vi "DAQ.vi"(0 "sample length":i32=100, 5 "task/channels in":refnum<k21>, 7 "SetVoltage":dbl=3.3 format="%#_13g", 9 "error in":errorcluster, 11 "VISA resource name out":refnum<visa-resource-name>, 12 "error out":errorcluster) -> (4 "task out":refnum<k21>, 6 "error out 2":errorcluster, 10 "VISA resource name out 2":refnum<visa-resource-name>, 15 "error out 3":errorcluster)   [LabVIEW 2018]
uses:
  <vilib>/DAQmx/read.llb/DAQmx Read (Analog DBL 1Chan 1Samp).vi
  GlobalVariables/GlobalStop.vi
  GlobalVariables/SetVoltagGlobal.vi
  GlobalVariables/Voltage Level Global.vi
  GlobalVariables/CurrentLevelGlobal.vi
  <vilib>/DAQmx/miscellaneous.llb/DAQmx Fill In Error Info.vi
  GlobalVariables/WaveformCharGlobal.vi
  <vilib>/ptbypt/NI_PtbyPt.lvlib
  OriginalCodeFolder/C/Program Files (x86)/National Instruments/LabVIEW 2018/instr.lib/XP Power PLS600/XP Power PLS600.lvlib
panel:
  in  "Over Voltage\nProtection":dbl=300.0 format="%#_13g"
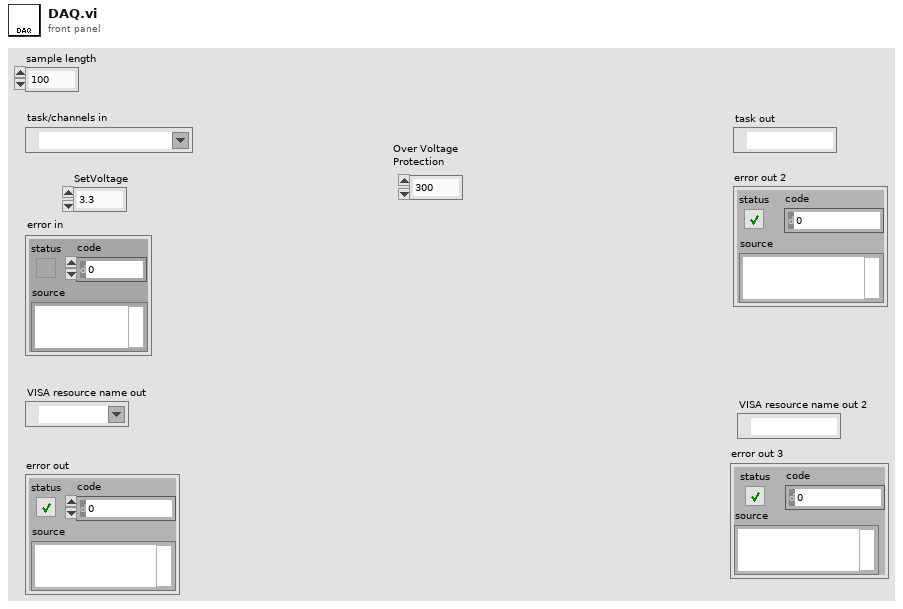
[diagram p1: front panel]
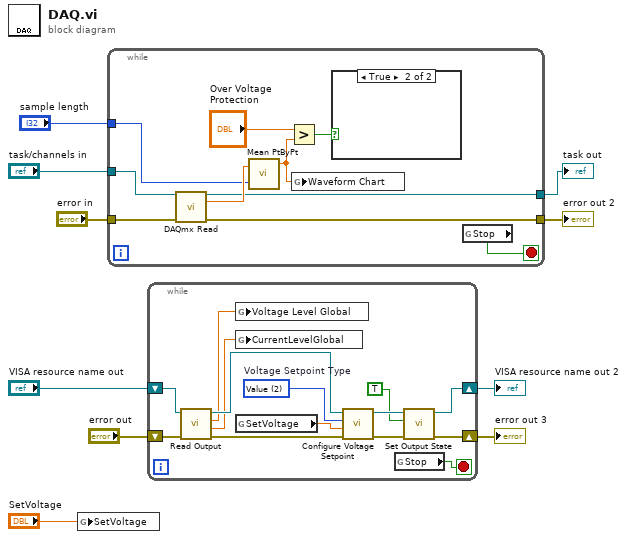
[diagram p0: block diagram]
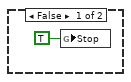
[diagram p2: hidden frame]
diagram:
  n1 = global write "SetVoltagGlobal.vi" "SetVoltage"("SetVoltage") -> ()
  n2 = while {
    tunnel: "sample length" -> [w14]
    tunnel: "task/channels in" -> [w13]
    tunnel: [w19] -> w3
    tunnel: "error in" -> [w12]
    tunnel: [w18] -> w4
    stop <- w15 stop-if-true
    n3 = call-poly <vilib>:"DAQmx Read.vi"("task/channels in"=w13, "error in"=w12) -> ("task out"=w19:refnum<k21>, "data"=w20:dbl, "error out"=w18:errorcluster)  [unwired: 11 in]
    n4 = call <vilib>:"Mean PtByPt.vi"("x"=w20, "sample length"=w14) -> ("mean"=w11:dbl)  [unwired: 2 in, 1 out]
    n5 = Greater?(x="Over Voltage\nProtection", y=w11) -> (0:w17:bool)
    n6 = global write "WaveformCharGlobal.vi" "Waveform Chart"(w11) -> ()
    n7 = case shown="True" w17 {
      frame False {
        n8 = global write "GlobalStop.vi" "Stop"(TRUE ("Over Allowable\nVoltage")) -> ()
      }
      frame True {
      }
    }
    n9 = global read "GlobalStop.vi" "Stop"() -> (w15:bool)
  }
  "error out 2" <- w4
  "task out" <- w3
  n10 = while {
    shift-right: [w31] -> w1
    shift-left: "error out" -> [w29]
    shift-right: [w30] -> w2
    shift-left: "VISA resource name out" -> [w27]
    stop <- w25 stop-if-true
    w33 = 2 items=["Minimum", "Maximum", "Value"]  # Voltage Setpoint Type
    n11 = call "Read Output.vi"("error in (no error)"=w29, "VISA resource name"=w27) -> ("error out"=w28:errorcluster, "Actual Current Level (amperes)"=w22:dbl, "Actual Voltage Level (volts)"=w23:dbl, "VISA resource name out"=w26:refnum<visa-resource-name>)  [unwired: 6 in]
    n12 = global write "Voltage Level Global.vi" "Voltage Level Global"(w23) -> ()
    n13 = global write "CurrentLevelGlobal.vi" "CurrentLevelGlobal"(w22) -> ()
    n14 = global read "SetVoltagGlobal.vi" "SetVoltage"() -> (w24:dbl)
    n15 = call "Configure Voltage Setpoint.vi"("error in (no error)"=w28, "Voltage Setpoint (0 volts)"=w24, "Voltage Setpoint Type (0: Minimum)"=w33, "VISA resource name"=w26) -> ("error out"=w34:errorcluster, "VISA resource name out"=w35:refnum<visa-resource-name>)  [unwired: 6 in]
    n16 = global read "GlobalStop.vi" "Stop"() -> (w25:bool)
    n17 = call "Set Output State.vi"("error in (no error)"=w34, "Output State (F: Disable)"=TRUE, "VISA resource name"=w35) -> ("error out"=w31:errorcluster, "VISA resource name out"=w30:refnum<visa-resource-name>)  [unwired: 7 in]
  }
  "VISA resource name out 2" <- w2
  "error out 3" <- w1
